vi "init.vi"(0 "EXC4Test in":refnum<class "EXC4Test.lvclass">, 1 "Tolerance":dbl[unit], 5 "Log":refnum<class "ITestLog.lvclass">, 7 "DAQ Channel To Read":refnum<k21>, 9 "Expected Value":dbl[unit], 11 "error in (no error)":errorcluster, 12 "Samples To Read":dbl) -> (4 "EXC4Test out":refnum<class "EXC4Test.lvclass">, 15 "error out":errorcluster)   [LabVIEW 2015, in "EXC4Test.lvclass"]
uses:
  EXC4Test.lvclass
  Model/TestLog/ITestLog/ITestLog.lvclass
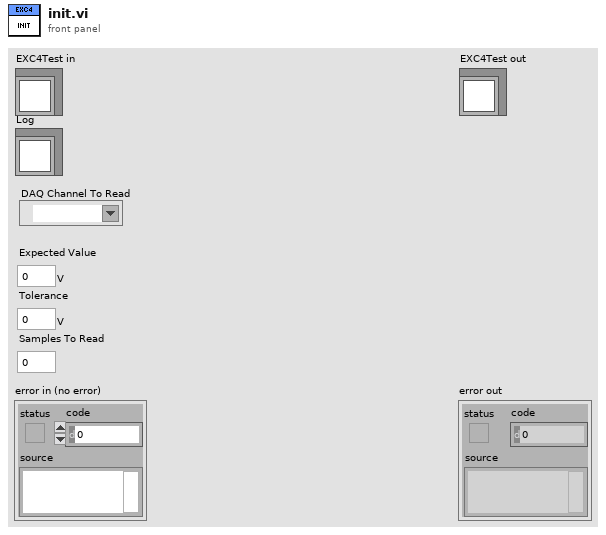
[diagram p1: front panel]
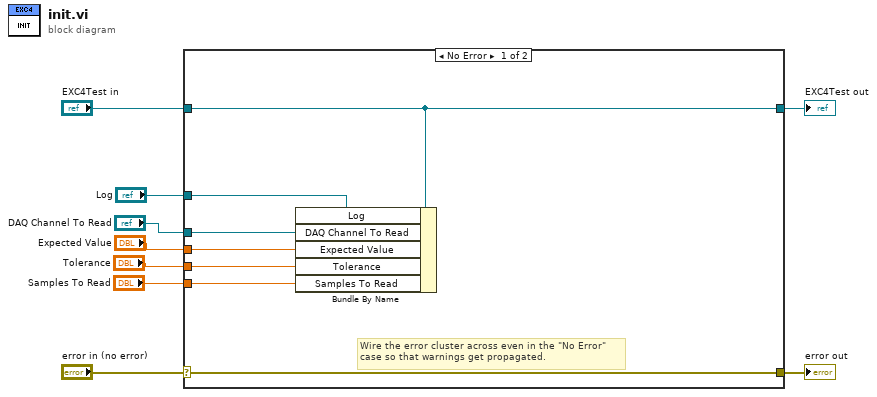
[diagram p0: block diagram]
diagram:
  n1 = case shown="No Error" "error in (no error)" {
    selector: "error in (no error)" -> [w16 w18]
    tunnel: [w16 w18] -> w8
    tunnel: [w14 w17] -> w6
    tunnel: "EXC4Test in" -> [w14 w17]
    tunnel: "Log" -> [w15 _]
    tunnel: "DAQ Channel To Read" -> [w13 _]
    tunnel: "Expected Value" -> [w12 _]
    tunnel: "Tolerance" -> [w11 _]
    tunnel: "Samples To Read" -> [w10 _]
    frame No Error {
      # "Wire the error cluster across even in the \"No Error\"\ncase so that warnings get propagated."
      n2 = Bundle By Name(cluster=w14, "Log"=w15, "DAQ Channel To Read"=w13, "Expected Value"=w12, "Tolerance"=w11, "Samples To Read"=w10) -> ()  [unwired: 1 out]
    }
    frame Error {
    }
  }
  "error out" <- w8
  "EXC4Test out" <- w6
